vi "ma_basicErrorCode2ErrorCluster.vi"(1 "error in (no error)":errorcluster caption="Fehler (Eingang, kein Fehler)", 2 "subVI name":string caption="SubVI-Name", 3 "Error Code":i32 caption="Fehlercode") -> (0 "error out":errorcluster caption="Fehler (Ausgang)")   [LabVIEW 2009]
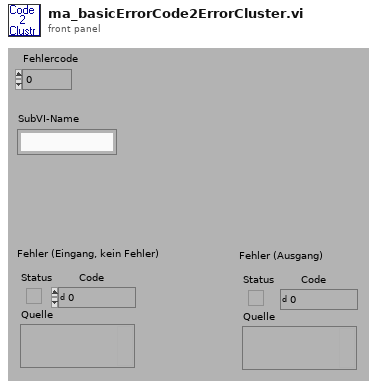
[diagram p1: front panel]
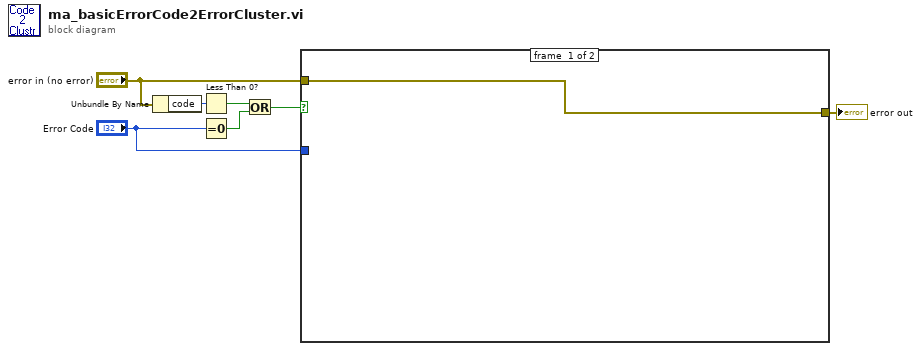
[diagram p0: block diagram]
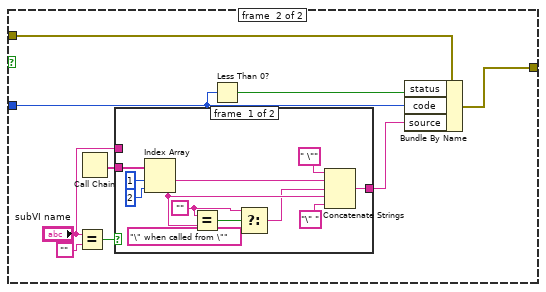
[diagram p2: hidden frame]
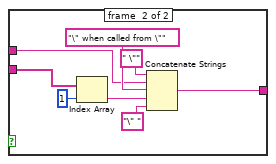
[diagram p3: hidden frame]
diagram:
  n1 = Unbundle By Name("error in (no error)") -> ("code"=w4:i32)
  n2 = Less Than 0?(x=w4) -> (x < 0?=w2:bool)
  n3 = Equal To 0?(x="Error Code") -> (x = 0?=w1:bool)
  n4 = Or(x=w2, y=w1) -> (x .or. y?=w3:bool)
  n5 = case shown="False" w3 {
    tunnel: "Error Code" -> [_ w14]
    tunnel: "error in (no error)" -> [w8 w17]
    tunnel: [w8 w16] -> w7
    frame #0 {
    }
    frame #1 {
      n6 = Equal?(x="subVI name", y="") -> (x = y?=w10:bool)
      n7 = Call Chain() -> (call chain=w11:string[])
      n8 = case shown="True" w10 {
        tunnel: [w24 w33] -> w15
        tunnel: w11 -> [w23 w32]
        tunnel: "subVI name" -> [_ w30]
        frame #0 {
          w20 = ""
          n9 = Index Array(array=w23, index #1=1 ("Index"), index #2=2 ("Index")) -> (element #1=w27:string, element #2=w21:string)
          n10 = Equal?(x=w20, y=w21) -> (x = y?=w22:bool)
          n11 = Select(t=w20, s=w22, f="\" when called from \"") -> (s? t:f=w18:string)
          n12 = Concatenate Strings(" \"" ("Substring"), w27, w18, w21, "\" ") -> (w24:string)
        }
        frame #1 {
          n13 = Index Array(array=w32, index=1 ("Index")) -> (element=w31:string)
          n14 = Concatenate Strings(" \"" ("Substring"), w30, "\" when called from \"", w31, "\" ") -> (w33:string)
        }
      }
      n15 = Less Than 0?(x=w14) -> (x < 0?=w13:bool)
      n16 = Bundle By Name(cluster=w17, "status"=w13, "code"=w14, "source"=w15) -> (w16:errorcluster)
    }
  }
  "error out" <- w7
